vi "speed control setting.vi"() -> ()   [LabVIEW 2019]
uses:
  database.lvlib
panel:
  in  "Error in 2":errorcluster
  out "Error out":errorcluster
  in  "Error THR":dbl=1.5 caption="Max. Speed (RPM)" min=0.5 max=3.0 step=0.25
  in  "Close":bool
  in  "Max. Speed (RPM)":dbl=5.5 min=5.0 max=6.0 step=0.1
  in  "Min. Speed (RPM)":dbl=3.2 min=3.0 max=4.0 step=0.1
  in  "pulse period (sec)":dbl=300.0 caption="Speed Control" min=180.0 max=600.0
  in  "Disc 30":dbl=12.5 min=11.0 max=13.0 step=0.1
  in  "Disc 29":dbl=12.5 min=11.0 max=13.0 step=0.1
  in  "Disc 28":dbl=12.5 min=11.0 max=13.0 step=0.1
  in  "Disc 27":dbl=12.5 min=11.0 max=13.0 step=0.1
  in  "Disc 26":dbl=12.5 caption="Set Point" min=10.0 max=13.0 step=0.1
  out "Name":string
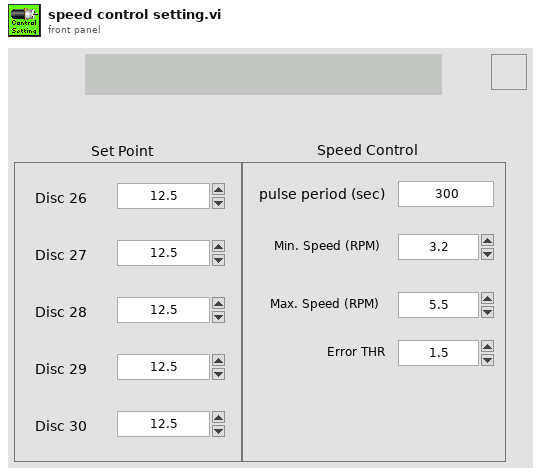
[diagram p1: front panel]
types:
  T1 = cluster{"Disc 26":dbl, "Disc 27":dbl, "Disc 28":dbl, "Disc 29":dbl, "Disc 30":dbl, "pulse period (sec)":dbl, "Max. Speed (RPM)":dbl, "Min. Speed (RPM)":dbl, "Error THR":dbl}
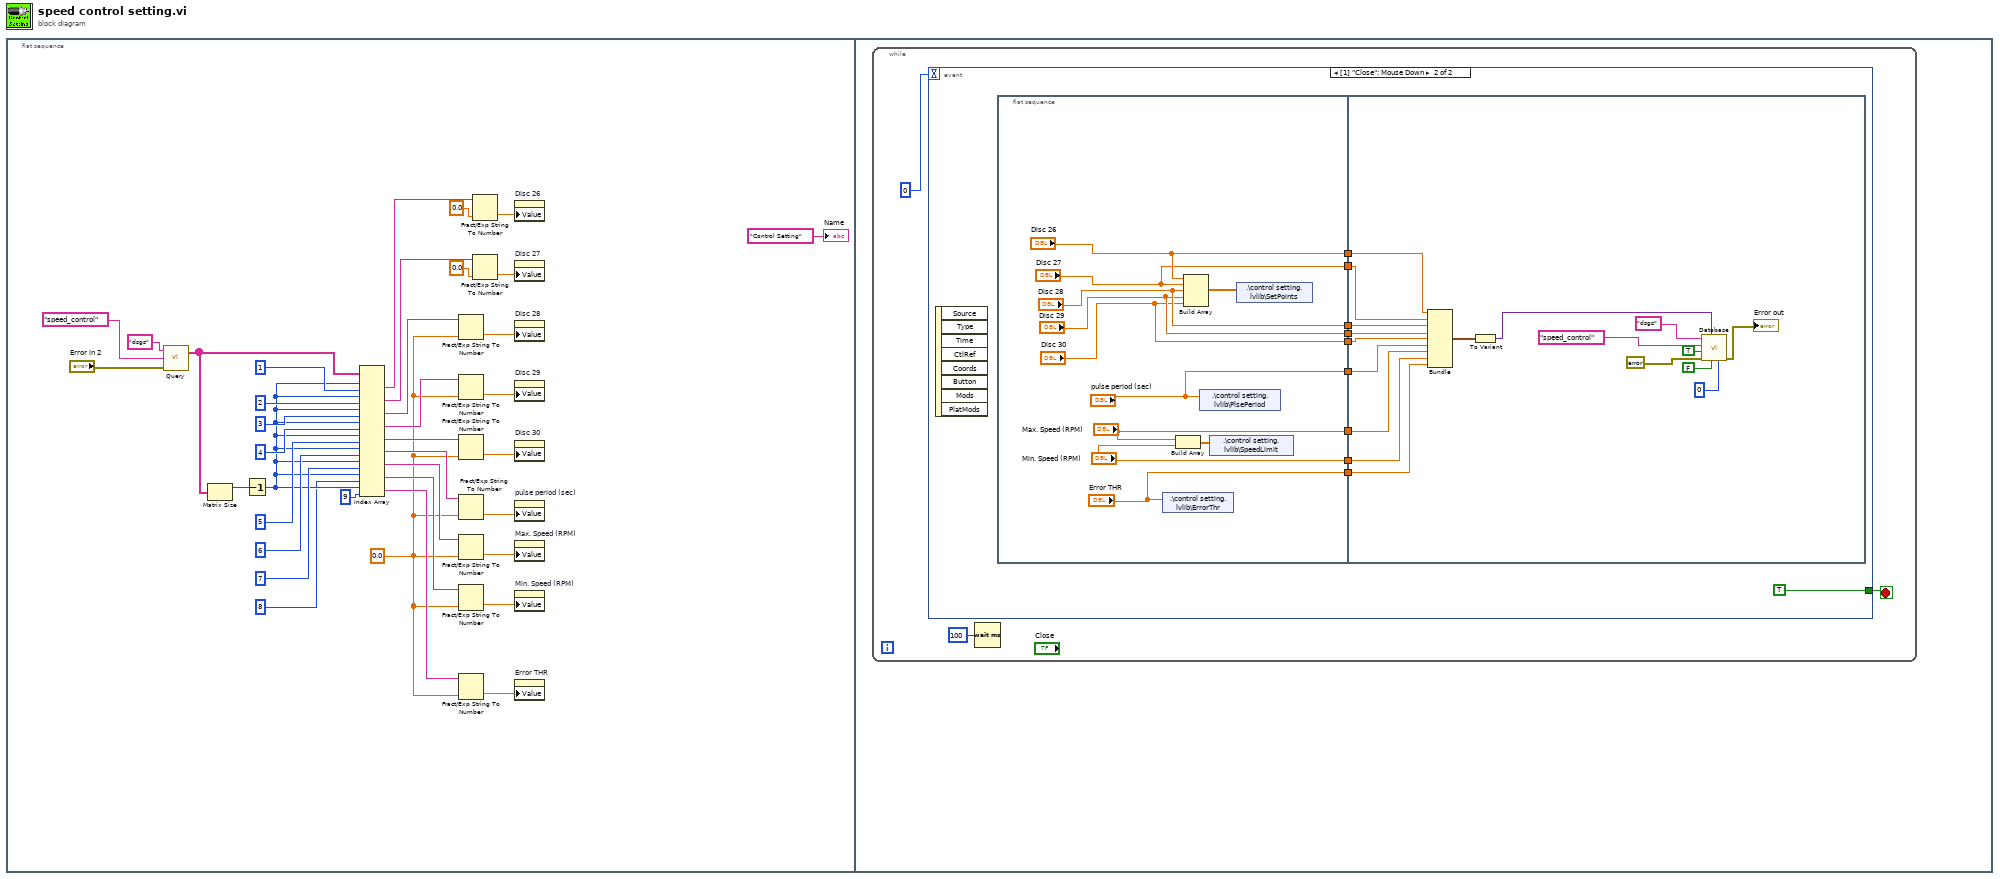
[diagram p0: block diagram]
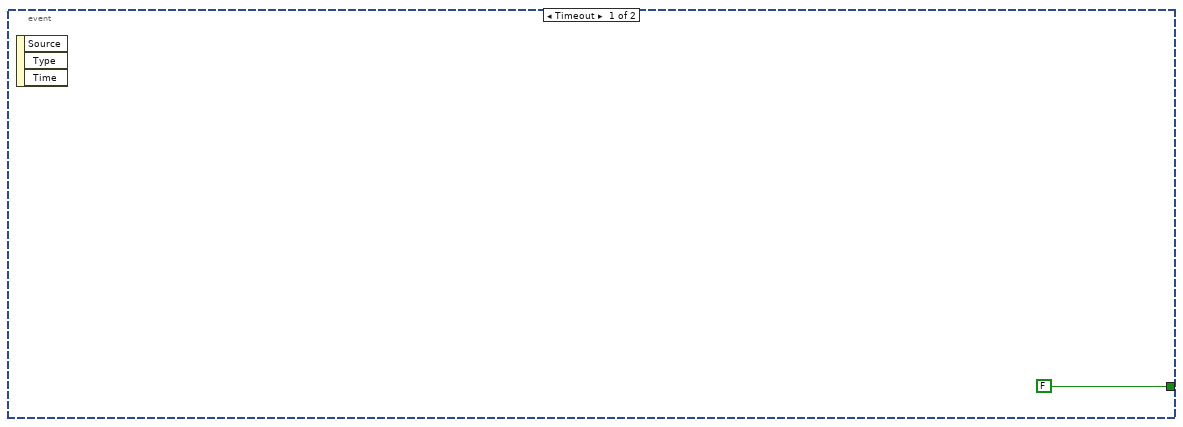
[diagram p2: hidden frame]
diagram:
  n1 = flat-sequence {
    frame #0 {
      w9 = 0.0 ("default (0 DBL)")
      n2 = call "Query.vi"("Error in"="Error in 2", "Table Name"="speed_control", "Connection Name"="dsgs") -> ("data"=w14:string[][])  [unwired: 1 in, 1 out]
      n3 = Matrix Size(0:w14) -> (1:w33:i32)  [unwired: 1 out]
      n4 = Decrement(x=w33) -> (x-1=w25:i32)
      n5 = Index Array(array=w14, index (row) #1=w25, index (col) #1=1 ("disabled index (col)"), index (row) #2=w25, index (col) #2=2 ("disabled index (col)"), index (row) #3=w25, index (col) #3=3 ("disabled index (col)"), index (row) #4=w25, index (col) #4=4 ("disabled index (col)"), index (row) #5=w25, index (col) #5=5 ("disabled index (col)"), index (row) #6=w25, index (col) #6=6 ("disabled index (col)"), index (row) #7=w25, index (col) #7=7 ("disabled index (col)"), index (row) #8=w25, index (col) #8=8 ("disabled index (col)"), index (row) #9=w25, index (col) #9=9 ("disabled index (col)")) -> (element #1=w22:string, element #2=w18:string, element #3=w17:string, element #4=w16:string, element #5=w15:string, element #6=w13:string, element #7=w12:string, element #8=w11:string, element #9=w10:string)
      n6 = Fract/Exp String To Number(string=w17, default (0 dbl)=w9) -> (number=w7:dbl)  [unwired: 2 in, 1 out]
      n7 = Fract/Exp String To Number(string=w16, default (0 dbl)=w9) -> (number=w6:dbl)  [unwired: 2 in, 1 out]
      n8 = Fract/Exp String To Number(string=w15, default (0 dbl)=w9) -> (number=w5:dbl)  [unwired: 2 in, 1 out]
      n9 = Fract/Exp String To Number(string=w13, default (0 dbl)=w9) -> (number=w4:dbl)  [unwired: 2 in, 1 out]
      n10 = Fract/Exp String To Number(string=w12, default (0 dbl)=w9) -> (number=w3:dbl)  [unwired: 2 in, 1 out]
      n11 = Fract/Exp String To Number(string=w11, default (0 dbl)=w9) -> (number=w2:dbl)  [unwired: 2 in, 1 out]
      n12 = Fract/Exp String To Number(string=w10, default (0 dbl)=w9) -> (number=w1:dbl)  [unwired: 2 in, 1 out]
      n13 = Fract/Exp String To Number(string=w22, default (0 dbl)=0.0 ("default (0 DBL)")) -> (number=w20:dbl)  [unwired: 2 in, 1 out]
      n14 = Fract/Exp String To Number(string=w18, default (0 dbl)=0.0 ("default (0 DBL)")) -> (number=w8:dbl)  [unwired: 2 in, 1 out]
      n15 = property on="Disc 26" class="DigNum (strict)"("Value"=w20) -> ()  [unwired: 2 in, 2 out]
      n16 = property on="Disc 27" class="DigNum (strict)"("Value"=w8) -> ()  [unwired: 2 in, 2 out]
      n17 = property on="Disc 28" class="DigNum (strict)"("Value"=w7) -> ()  [unwired: 2 in, 2 out]
      n18 = property on="Disc 29" class="DigNum (strict)"("Value"=w6) -> ()  [unwired: 2 in, 2 out]
      n19 = property on="Disc 30" class="DigNum (strict)"("Value"=w5) -> ()  [unwired: 2 in, 2 out]
      n20 = property on="pulse period (sec)" class="DigNum (strict)"("Value"=w4) -> ()  [unwired: 2 in, 2 out]
      n21 = property on="Max. Speed (RPM)" class="DigNum (strict)"("Value"=w3) -> ()  [unwired: 2 in, 2 out]
      n22 = property on="Min. Speed (RPM)" class="DigNum (strict)"("Value"=w2) -> ()  [unwired: 2 in, 2 out]
      n23 = property on="Error THR" class="DigNum (strict)"("Value"=w1) -> ()  [unwired: 2 in, 2 out]
      "Name" <- "Control Setting" ("Name")
    }
    frame #1 {
      n24 = while {
        stop <- w39 stop-if-true
        n25 = event shown="[1] \"Close\": Mouse Down" {
          selector: _ -> [_ _]
          dyn-events: _ -> [_ _]
          timeout: 0 -> [_ _]
          tunnel: [FALSE TRUE] -> w39
          event Timeout {
            n26 = event-data() -> ()  [unwired: 1 in, 3 out]
          }
          event "Close": Mouse Down {
            n27 = event-data() -> ()  [unwired: 1 in, 8 out]
            n28 = flat-sequence {
              tunnel: ["Disc 26"] -> w50
              tunnel: ["Disc 27"] -> w49
              tunnel: ["Disc 28"] -> w48
              tunnel: ["Disc 29"] -> w47
              tunnel: ["Disc 30"] -> w46
              tunnel: ["pulse period (sec)"] -> w45
              tunnel: ["Max. Speed (RPM)"] -> w44
              tunnel: ["Min. Speed (RPM)"] -> w43
              tunnel: ["Error THR"] -> w42
              tunnel: w50 -> [w78]
              tunnel: w49 -> [w77]
              tunnel: w48 -> [w76]
              tunnel: w47 -> [w75]
              tunnel: w46 -> [w74]
              tunnel: w45 -> [w73]
              tunnel: w44 -> [w72]
              tunnel: w43 -> [w71]
              tunnel: w42 -> [w70]
              frame #0 {
                n29 = shared-variable ".\\control setting.lvlib\\ErrorThr"("Error THR") -> ()  [unwired: 1 in, 1 out]
                n30 = Build Array("Max. Speed (RPM)", "Min. Speed (RPM)") -> (w61:dbl[])
                n31 = Build Array("Disc 26", "Disc 27", "Disc 28", "Disc 29", "Disc 30") -> (w62:dbl[])
                n32 = shared-variable ".\\control setting.lvlib\\PlsePeriod"("pulse period (sec)") -> ()  [unwired: 1 in, 1 out]
                n33 = shared-variable ".\\control setting.lvlib\\SpeedLimit"(w61) -> ()  [unwired: 1 in, 1 out]
                n34 = shared-variable ".\\control setting.lvlib\\SetPoints"(w62) -> ()  [unwired: 1 in, 1 out]
              }
              frame #1 {
                n35 = Bundle("Disc 26"=w78, "Disc 27"=w77, "Disc 28"=w76, "Disc 29"=w75, "Disc 30"=w74, "pulse period (sec)"=w73, "Max. Speed (RPM)"=w72, "Min. Speed (RPM)"=w71, "Error THR"=w70) -> (w69:T1)  [unwired: 1 in]
                n36 = To Variant(anything=w69) -> (Variant=w68:variant)
                n37 = call "Database.vi"("Maximum Row"=0, "Delete row?"=FALSE, "Data"=w68, "Error in"=errorcluster {"status"=FALSE, "code"=0, "source"=""}, "Auto Increment ID?"=TRUE, "Table"="speed_control", "Connection"="dsgs") -> ("Error out"=→"Error out":errorcluster)  [unwired: 4 in]
              }
            }
          }
        }
        n38 = Wait (ms)(milliseconds to wait=u32 100) -> ()  [unwired: 1 out]
      }
    }
  }
